vi "local_orientation.vi"(11 "目标位置":dbl[](array[numeric])) -> (3 "Array":dbl[][](array[numeric]))   [LabVIEW 2017]
uses:
  <vilib>/Analysis/NI_AALPro.lvlib
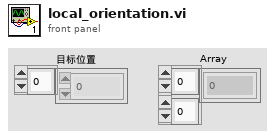
[diagram p1: front panel]
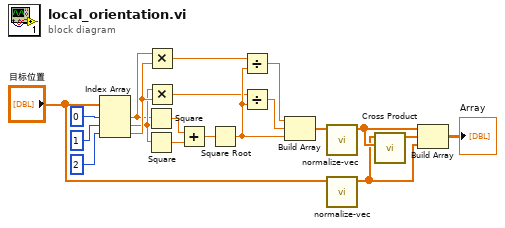
[diagram p0: block diagram]
diagram:
  n1 = Index Array(array="目标位置", index #1=0 ("index"), index #2=1 ("index"), index #3=2 ("index")) -> (element #1=w8:dbl, element #2=w11:dbl, element #3=w12:dbl)
  n2 = Square(x=w8) -> (x^2=w5:dbl)
  n3 = Square(x=w11) -> (x^2=w6:dbl)
  n4 = Multiply(x=w8, y=w12) -> (x*y=w9:dbl)
  n5 = Multiply(x=w11, y=w12) -> (x*y=w13:dbl)
  n6 = Add(x=w5, y=w6) -> (x+y=w7:dbl)
  n7 = Square Root(x=w7) -> (sqrt(x)=w14:dbl)
  n8 = Divide(x=w9, y=w14) -> (x/y=w10:dbl)
  n9 = Divide(x=w13, y=w14) -> (x/y=w15:dbl)
  n10 = Build Array(w10, w15, w14) -> (w16:dbl[])
  n11 = call "normalize-vec.vi"("Vec Input"=w16) -> ("Array Output"=w18:dbl[])  [unwired: 7 in, 3 out]
  n12 = call "normalize-vec.vi"("Vec Input"="目标位置") -> ("Array Output"=w17:dbl[])  [unwired: 7 in, 3 out]
  n13 = call <vilib>:"Cross Product.vi"("B Vector"=w18, "A Vector"=w17) -> ("Cross Product"=w19:dbl[])  [unwired: 8 in, 1 out]
  n14 = Build Array(w18, w19, w17) -> (→"Array":dbl[][])
